vi "Boolean Toggle.vi"(1 "Input":bool, 12 "Reset":bool) -> (21 "Output":bool)   [LabVIEW 2016]
doc: "Changes a standard boolean input to a toggled boolean output."
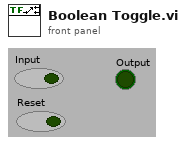
[diagram p1: front panel]
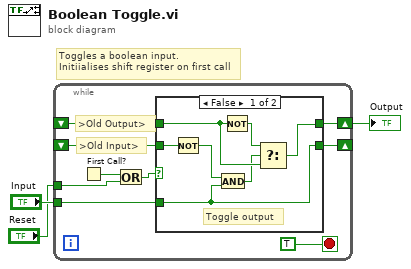
[diagram p0: block diagram]
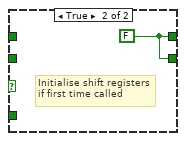
[diagram p2: hidden frame]
diagram:
  # "Toggles a boolean input.\nInitiialises shift register on first call"
  n1 = while {
    shift-right: [w12] -> w3
    shift-left: _ -> [w11]
    shift-right: [w7] -> _
    shift-left: _ -> [w9]
    tunnel: "Input" -> [w8]
    tunnel: "Reset" -> [w5]
    stop <- TRUE stop-if-true
    # ">Old Input>"
    # ">Old Output>"
    n2 = First Call?() -> (First Call?: T/F=w6:bool)
    n3 = Or(x=w6, y=w5) -> (x .or. y?=w4:bool)
    n4 = case shown="False" w4 {
      tunnel: [w18 w20] -> w12
      tunnel: w11 -> [w17 _]
      tunnel: w9 -> [w13 _]
      tunnel: w8 -> [w14 _]
      tunnel: [w14 w20] -> w7
      frame False {
        # "Toggle output"
        n5 = Not(x=w13) -> (.not. x?=w16:bool)
        n6 = And(x=w16, y=w14) -> (x .and. y?=w15:bool)
        n7 = Not(x=w17) -> (.not. x?=w19:bool)
        n8 = Select(t=w19, s=w15, f=w17) -> (s? t:f=w18:bool)
      }
      frame True {
        w20 = FALSE
        # "Initialise shift registers\nif first time called"
      }
    }
  }
  "Output" <- w3
